vi "Update Power.vi"(8 "error in (no error)":errorcluster, 10 "event data":cluster{"Label":string, "Value":dbl}, 11 "Laser Oxxius Controller in":refnum<class "Laser Oxxius Controller.lvclass">) -> (0 "error out":errorcluster, 3 "Laser Oxxius Controller out":refnum<class "Laser Oxxius Controller.lvclass">)   [LabVIEW 2020, in "Laser_Oxxius.lvlib" / "Laser Oxxius Controller.lvlib" / "Laser Oxxius Controller.lvclass"]
uses:
  Laser Oxxius Controller.lvclass
  Laser Oxxius Controller.lvclass/Laser Oxxius Controller.ctl
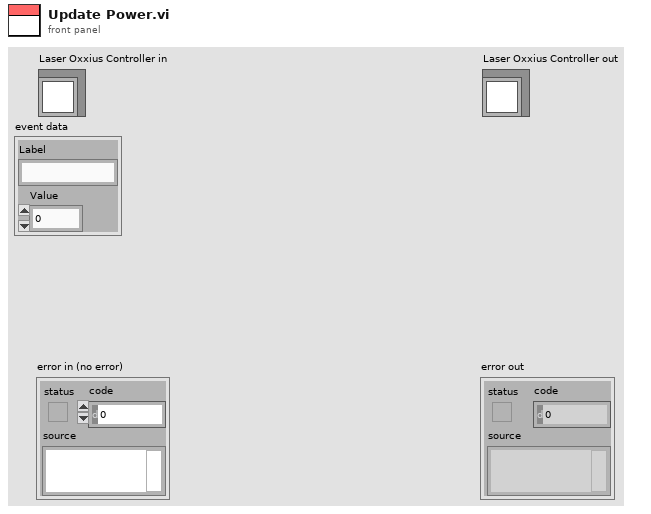
[diagram p1: front panel]
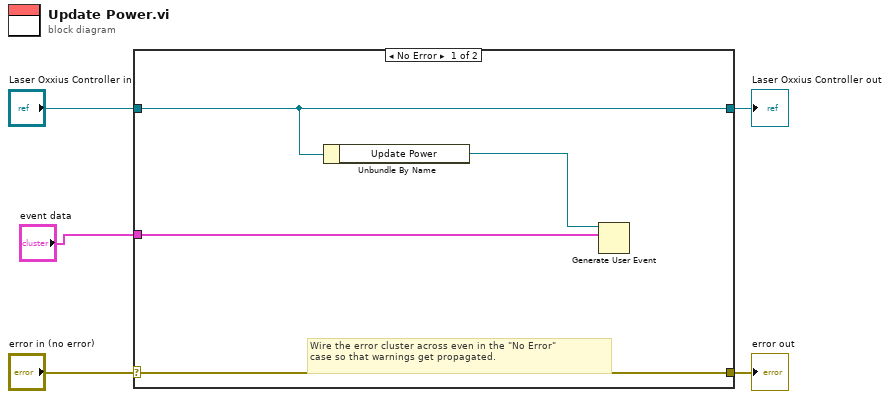
[diagram p0: block diagram]
diagram:
  n1 = case shown="No Error" "error in (no error)" {
    selector: "error in (no error)" -> [w9 w11]
    tunnel: [w9 w11] -> w4
    tunnel: [w7 w10] -> w2
    tunnel: "Laser Oxxius Controller in" -> [w7 w10]
    tunnel: "event data" -> [w6 _]
    frame No Error {
      # "Wire the error cluster across even in the \"No Error\"\ncase so that warnings get propagated."
      n2 = Unbundle By Name(w7) -> ("Update Power"=w8:refnum<user-event>)
      n3 = Generate User Event(user event=w8, event data cluster=w6) -> ()  [unwired: 2 in, 2 out]
    }
    frame Error {
    }
  }
  "error out" <- w4
  "Laser Oxxius Controller out" <- w2
